vi "PlotStates.vi"(5 "Width":u32, 7 "Height":u32, 8 "error in (no error)":errorcluster, 9 "XScale.Max":dbl, 11 "waveform in":waveform(dbl)) -> (0 "error out":errorcluster, 2 "Middle":picture, 3 "Back":picture)   [LabVIEW 2012, in "Report.lvlib"]
uses:
  Report.lvlib
  State.ctl
  <vilib>/Waveform/WDTOps.llb/WDT Get Final Time Value DBL.vi
  <vilib>/Waveform/WDTOps.llb/WDT Get XY Value DBL.vi
  <vilib>/Waveform/WDTOps.llb/WDT Number of Waveform Samples DBL.vi
panel:
  out "State":T1=enum."HUNTING"
  in  "rect":T2
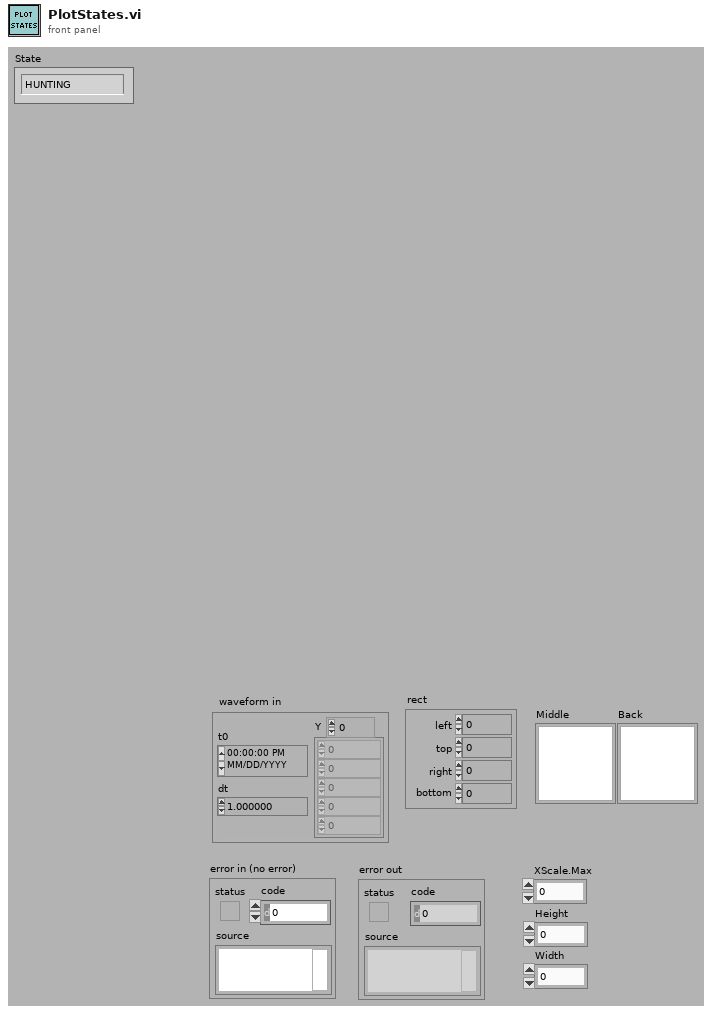
[diagram p1: front panel]
types:
  T1 = typedef "State.ctl" = enum16{"READY", "LOAD", "LOCALIZATION", "HUNTING", "SEAL", "BREAKIN", "WCR", "ALIGN", "APPROACH", "TARGETING"}
  T2 = cluster{"left":i16, "top":i16, "right":i16, "bottom":i16}
  T3 = cluster{"Font Name:":string, "Size":i16, "Strikeout?":bool, "Italic?":bool, "Underline?":bool, "Outline?":bool, "Shadow?":bool, "Bold?":bool}
  T4 = enum16{"User-specified Font", "Application Font", "System Font", "Dialog Font"}
  T5 = enum16{"None", "Stacked", "Clockwise", "Counterclockwise"}
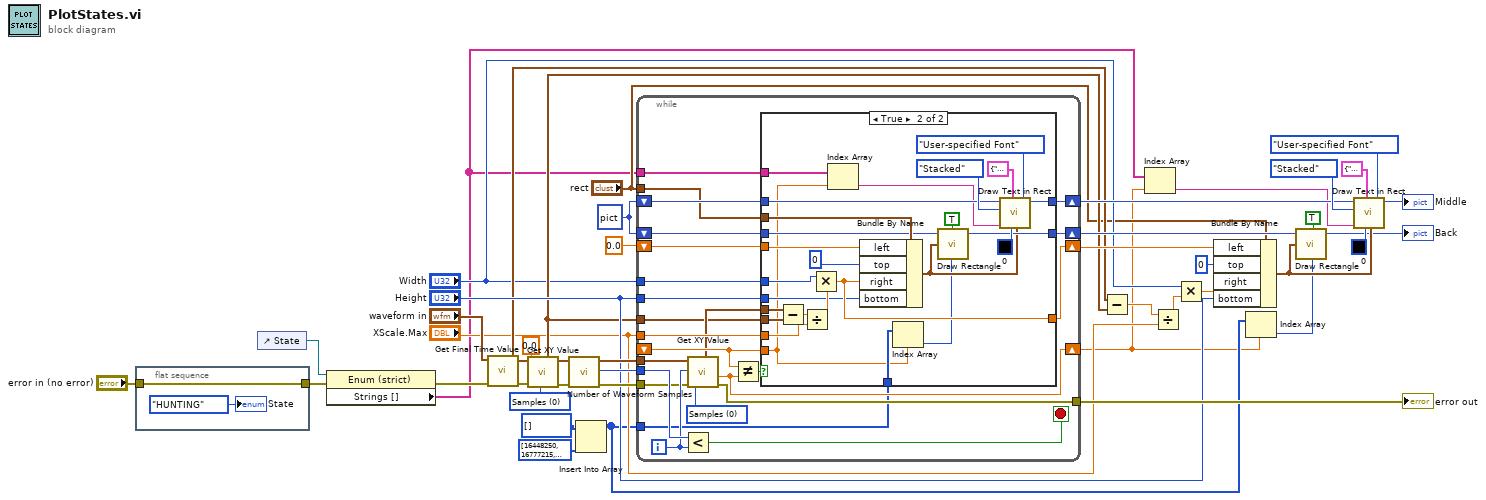
[diagram p0: block diagram]
diagram:
  w42 = u16 0 items=["Samples", "Relative Time"] ("Y position format")
  w39 = picture data[5B] ("picture")
  n1 = flat-sequence {
    tunnel: [w46] -> w5
    tunnel: "error in (no error)" -> [w46]
    frame #0 {
      "State" <- State."HUNTING" ("State")
    }
  }
  n2 = control-ref of="State"() -> (w7:refnum<vi>)
  n3 = property class="Enum (strict)"(reference=w7, error in=w5) -> (error out=w6:errorcluster, "Strings []"=w2:string[])  [unwired: 1 out]
  n4 = call-poly <vilib>:"Get Final Time Value.vi"("error in (no error)"=w6, "waveform in"="waveform in") -> ("error out"=w18:errorcluster, "tf"=w16:timestamp, "waveform out"=w17:waveform(dbl))  [unwired: 7 in]
  n5 = call-poly <vilib>:"Get XY Value.vi"("error in (no error)"=w18, "Y position"=0.0, "Y position format"=w42, "waveform in"=w17) -> ("error out"=w38:errorcluster, "waveform out"=w40:waveform(dbl), "X value"=w19:timestamp)  [unwired: 3 in, 2 out]
  n6 = call-poly <vilib>:"Number of Waveform Samples.vi"("error in (no error)"=w38, "waveform in"=w40) -> ("error out"=w37:errorcluster, "number of samples"=w44:i32, "waveform out"=w45:waveform(dbl))  [unwired: 7 in]
  n7 = Insert Into Array(array=u32[] [], new element=u32[] [16448250, 16777215, 15269887, 15400919, 16775133, 16774388, 16448250, 16251385, 16448250, 16448250, 16448250, 16448250, 16448250]) -> (w11:u32[])  [unwired: 1 in]
  n8 = while {
    tunnel: w45 -> [w71]
    tunnel: w44 -> [w65]
    shift-right: [w56] -> w3
    shift-left: _ -> [w58]
    shift-right: [w61] -> w24
    shift-left: w39 -> [w70]
    shift-right: [w68] -> w23
    shift-left: 0.0 -> [w60]
    tunnel: w19 -> [w53]
    shift-right: [w62] -> w25
    shift-left: w39 -> [w63]
    tunnel: "XScale.Max" -> [w55]
    tunnel: w37 -> [w59]
    tunnel: [w57] -> w36
    tunnel: "Width" -> [w52]
    tunnel: "Height" -> [w51]
    tunnel: w11 -> [w50]
    tunnel: "rect" -> [w49]
    tunnel: w2 -> [w48]
    i -> [w64]
    stop <- w69 stop-if-true
    w67 = u16 0 items=["Samples", "Relative Time"] ("Y position format")
    n9 = Less?(x=w65, y=w64) -> (x < y?=w69:bool)
    n10 = call-poly <vilib>:"Get XY Value.vi"("error in (no error)"=w59, "Y position"=w64, "Y position format"=w67, "waveform in"=w71) -> ("error out"=w57:errorcluster, "Y value"=w56:dbl, "X value"=w54:timestamp)  [unwired: 3 in, 2 out]
    n11 = Not Equal?(x=w58, y=w56) -> (x != y?=w66:bool)
    n12 = case shown="True" w66 {
      tunnel: w70 -> [w74 w81]
      tunnel: [w74 w82] -> w61
      tunnel: w60 -> [w73 w99]
      tunnel: [w73 w92] -> w68
      tunnel: w58 -> [_ w77]
      tunnel: w63 -> [w72 w84]
      tunnel: [w72 w98] -> w62
      tunnel: w55 -> [_ w96]
      tunnel: w54 -> [_ w94]
      tunnel: w53 -> [_ w93]
      tunnel: w52 -> [_ w90]
      tunnel: w51 -> [_ w89]
      tunnel: w50 -> [_ w86]
      tunnel: w49 -> [_ w85]
      tunnel: w48 -> [_ w76]
      frame False {
      }
      frame True {
        n13 = Subtract(x=w94, y=w93) -> (x-y=w95:dbl)
        n14 = Divide(x=w95, y=w96) -> (x/y=w91:dbl)
        n15 = Multiply(x=w90, y=w91) -> (x*y=w92:dbl)
        n16 = Index Array(array=w76, index=w77) -> (element=w75:string)
        n17 = Bundle By Name(cluster=w85, "left"=w99, "top"=i16 0, "right"=w92, "bottom"=w89) -> (w80:T2)
        n18 = Index Array(array=w86, index=w77) -> (element=w79:u32)
        n19 = call <vilib>:"Draw Rectangle.vi"("picture"=w81, "rect"=w80, "fill?(F)"=TRUE, "color(black)"=w79) -> ("new picture"=w82:picture)  [unwired: 5 in]
        n20 = call <vilib>:"Draw Text in Rect.vi"("[user-specified font]"=T3 {"Font Name:"="x", "Size"=12, "Strikeout?"=FALSE, "Italic?"=FALSE, "Underline?"=FALSE, "Outline?"=FALSE, "Shadow?"=FALSE, "Bold?"=FALSE}, "text color(black)"=u32 0, "desired font(Application)"=T4."User-specified Font", "text"=w75, "rect"=w80, "text orientation"=T5."Stacked", "picture"=w84) -> ("new picture"=w98:picture)  [unwired: 4 in]
      }
    }
  }
  "error out" <- w36
  n21 = Subtract(x=w16, y=w19) -> (x-y=w31:dbl)
  n22 = Index Array(array=w2, index=w3) -> (element=w1:string)
  n23 = Divide(x=w31, y="XScale.Max") -> (x/y=w29:dbl)
  n24 = Multiply(x="Width", y=w29) -> (x*y=w30:dbl)
  n25 = Bundle By Name(cluster="rect", "left"=w23, "top"=i16 0, "right"=w30, "bottom"="Height") -> (w34:T2)
  n26 = Index Array(array=w11, index=w3) -> (element=w10:u32)
  n27 = call <vilib>:"Draw Rectangle.vi"("picture"=w24, "rect"=w34, "fill?(F)"=TRUE, "color(black)"=w10) -> ("new picture"=→"Back":picture)  [unwired: 5 in]
  n28 = call <vilib>:"Draw Text in Rect.vi"("[user-specified font]"=T3 {"Font Name:"="x", "Size"=12, "Strikeout?"=FALSE, "Italic?"=FALSE, "Underline?"=FALSE, "Outline?"=FALSE, "Shadow?"=FALSE, "Bold?"=FALSE}, "text color(black)"=u32 0, "desired font(Application)"=T4."User-specified Font", "text"=w1, "rect"=w34, "text orientation"=T5."Stacked", "picture"=w25) -> ("new picture"=→"Middle":picture)  [unwired: 4 in]
